vi "visa_write.vi"() -> ()   [LabVIEW 2016]
uses:
  <vilib>/Instr/_visa.llb/VISA Configure Serial Port (Instr).vi
panel:
  in  "写入缓冲区":string
  in  "串口配置":T1 {"数据位" items=["8"=8]; "流控制" items=["无"=0, "XON/XOFF"=1, "RTS/CTS"=2, "DTR/DSR"=4]; "停止位" items=["1.0"=10, "2.0"=15, "3.0"=20]; "奇偶校验位" items=["None"]; "波特率" items=["115200"=115200]}
  in  "VISA资源名称":refnum<visa-resource-name>
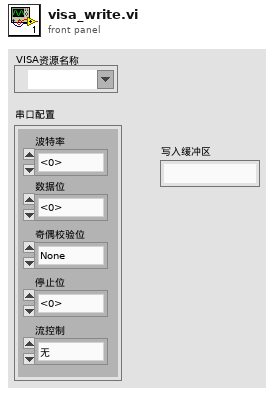
[diagram p1: front panel]
types:
  T1 = cluster{"波特率":u32, "奇偶校验位":u16, "停止位":u16, "流控制":u16, "数据位":u32}
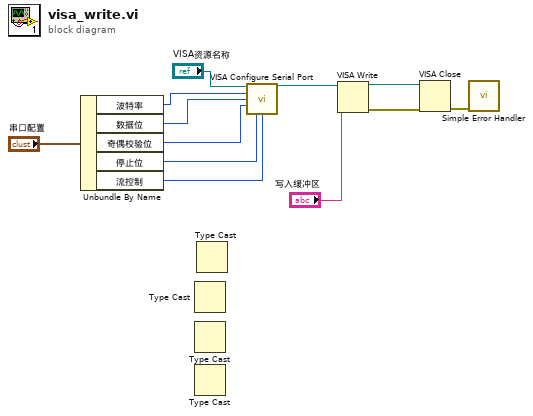
[diagram p0: block diagram]
diagram:
  n1 = Unbundle By Name("串口配置") -> ("波特率"=w9:u32, "数据位"=w8:u32, "奇偶校验位"=w7:u16, "停止位"=w6:u16, "流控制"=w5:u16)
  n2 = Type Cast() -> ()  [unwired: 2 in, 1 out]
  n3 = Type Cast() -> ()  [unwired: 2 in, 1 out]
  n4 = Type Cast() -> ()  [unwired: 2 in, 1 out]
  n5 = Type Cast() -> ()  [unwired: 2 in, 1 out]
  n6 = call-poly "VISA Configure Serial Port"("VISA resource name"="VISA资源名称", "baud rate (9600)"=w9, "data bits (8)"=w8, "parity (0:none)"=w7, "stop bits (10: 1 bit)"=w6, "flow control (0:none)"=w5) -> ("VISA resource name out"=w4:refnum<visa-resource-name>)  [unwired: 8 in, 1 out]
  n7 = VISA Write(VISA resource name=w4, write buffer="写入缓冲区") -> (VISA resource name out=w2:refnum<visa-resource-name>, error out=w3:errorcluster)  [unwired: 1 in, 1 out]
  n8 = VISA Close(VISA resource name=w2, error in (no error)=w3) -> (error out=w11:errorcluster)
  n9 = call <vilib>:"Simple Error Handler.vi"("error in (no error)"=w11) -> ()  [unwired: 4 in, 5 out]
